vi "Analyze ball (SubVI).vi"(0 "ROI Descriptor COLOR Mask":T2={"Global Rectangle"=[109, 72, 345, 284], "Contours"=[{"ID"=enum."External", "Type"=3, "Coordinates"=[109, 72, 345, 284]}]} {"Contours"."Type" items=["No Selection", "Point", "Line", "Rectangle", "Oval", "Polygon", "Freehand Region", "Annulus", "Unused2", "Unused3", "Broken Line", "Freehand Line", "Rotated Rectangle"]}, 1 "Radius":dbl, 2 "Boolean":bool, 3 "curX":dbl, 4 "curY":dbl, 5 "divider (circle)":dbl=1.0, 6 "Image In":T1, 7 "error in":errorcluster) -> (11 "Color":i32, 12 "Image Out":T1, 13 "error out":errorcluster, 14 "ROI Descriptor COLOR Mask out":T2={"Global Rectangle"=[109, 72, 345, 284], "Contours"=[{"ID"=enum."External", "Type"=3, "Coordinates"=[109, 72, 345, 284]}]} {"Contours"."Type" items=["No Selection", "Point", "Line", "Rectangle", "Oval", "Polygon", "Freehand Region", "Annulus", "Unused2", "Unused3", "Broken Line", "Freehand Line", "Rotated Rectangle"]}, 15 "x0":i32, 16 "y0":i32, 17 "x1":i32, 18 "y1":i32)   [LabVIEW 2017]
uses:
  <vilib>/vision/Image Controls.llb/IMAQ Image.ctl
panel:
  # "img out"
  # "img in"
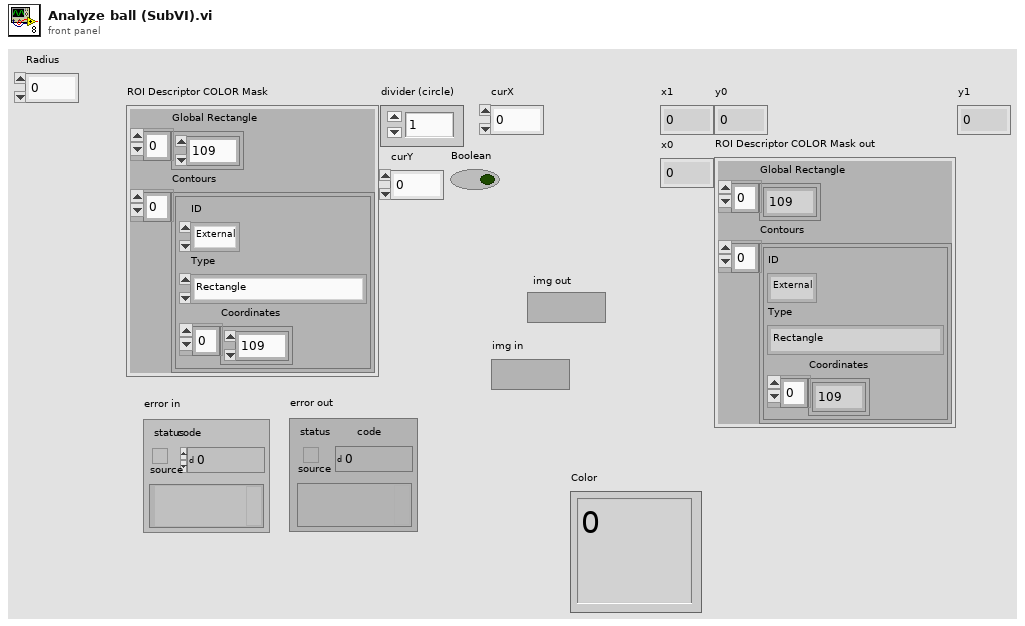
[diagram p1: front panel]
types:
  T1 = typedef "IMAQ Image.ctl" = refnum<image>
  T2 = cluster{"Global Rectangle":i32[], "Contours":cluster{"ID":enum32{"External", "Internal"}, "Type":u32, "Coordinates":i32[]}[]}
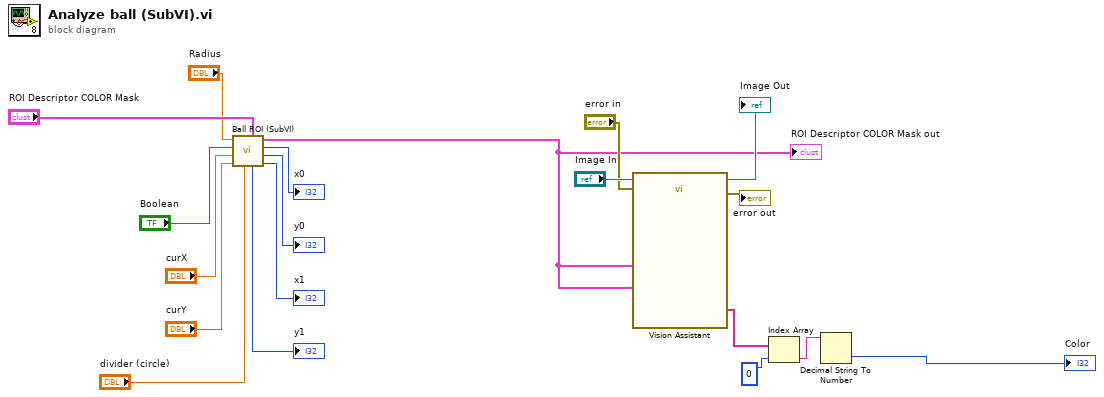
[diagram p0: block diagram]
diagram:
  n1 = call "Ball ROI (SubVI).vi"("ROI Descriptor COLOR Mask"="ROI Descriptor COLOR Mask", "divider (circle)"="divider (circle)", "curY"="curY", "curX"="curX", "Boolean"="Boolean", "Radius"="Radius") -> ("x1"=→"x1":i32, "y0"=→"y0":i32, "x0"=→"x0":i32, "ROI Descriptor COLOR Mask out"=w2:T2, "y1"=→"y1":i32)  [unwired: 1 in]
  "ROI Descriptor COLOR Mask out" <- w2
  n2 = call "Vision Assistant"("Image In"="Image In", "error in"="error in", "ROI Descriptor (Image Mask 1)"=w2, "ROI Descriptor (Color Classification 1)"=w2) -> ("Image Out"=→"Image Out":T1, "error out"=→"error out":errorcluster, "Classes (Color Classification 1)"=w4:string[])  [unwired: 21 in]
  n3 = Index Array(array=w4, index=0) -> (element=w6:string)
  n4 = Decimal String To Number(string=w6) -> (number=→"Color":i32)  [unwired: 2 in, 1 out]
